vi "CFTS-Init State.vi"(9 "Root folder":path, 10 "CFTS Version":string, 11 "Experiment State (in)":T1) -> (0 "error out":errorcluster, 3 "Experiment State (out)":T1)   [LabVIEW 2020]
doc: "Initializes ABI experiment state based on the specified experiment ID."
uses:
  CFTS-Experiment State.ctl
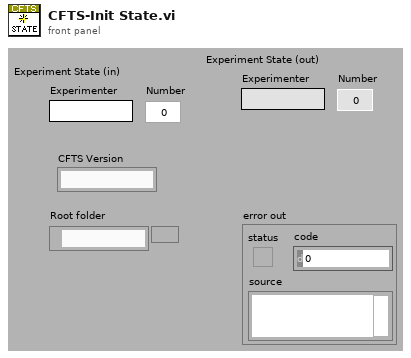
[diagram p1: front panel]
types:
  T1 = typedef "CFTS-Experiment State.ctl" = cluster{"Experimenter":string, "Number":u32, "Right":string, "Left":string, "Data Folder":path, "State File":path, "Version Info":string, "End Exposure Time":dbl, "Exposure Duration":string, "Run #":cluster{"CAP":i16, "ABR":i16, "DP":i16, "VsEP":i16, "MeasSeq":i16, "SubSeq":i16, "SFOAE":i16}}
  T2 = cluster{"CAP":i16, "ABR":i16, "DP":i16, "VsEP":i16, "MeasSeq":i16, "MeasSeq 2":i16, "MeasSeq 3":i16}
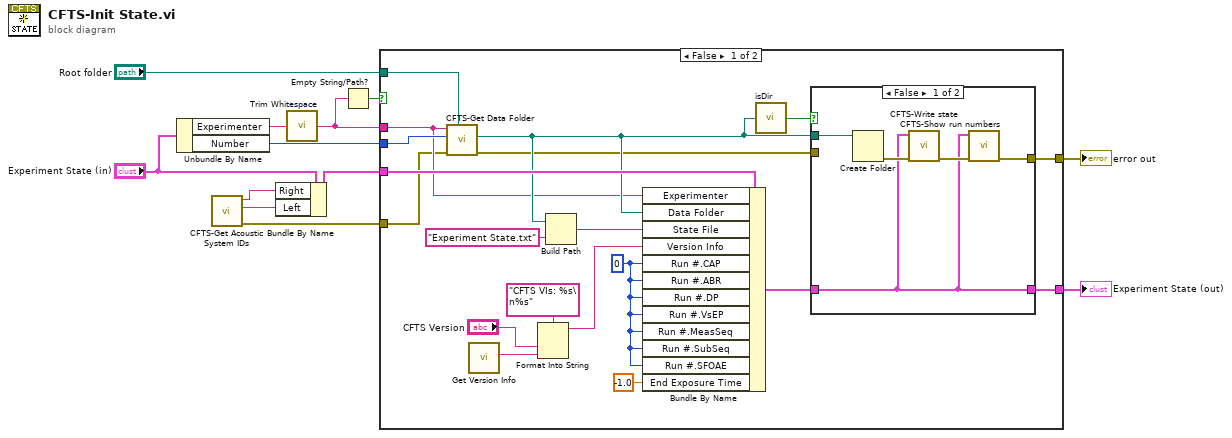
[diagram p0: block diagram]
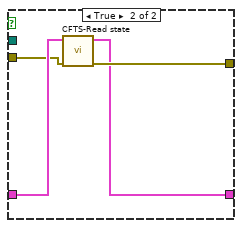
[diagram p2: hidden frame]
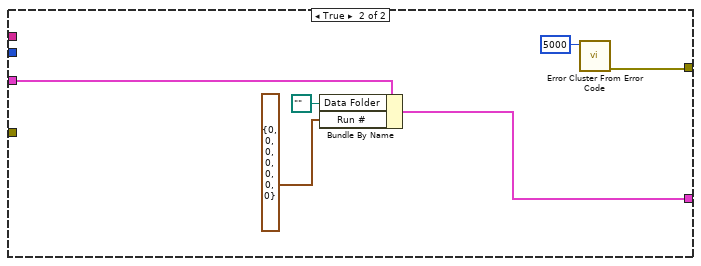
[diagram p3: hidden frame]
diagram:
  n1 = Unbundle By Name("Experiment State (in)") -> ("Experimenter"=w9:string, "Number"=w12:u32)
  n2 = call "CFTS-Get Acoustic System IDs.vi"() -> ("error out"=w2:errorcluster, "Left"=w6:string, "Right"=w5:string)  [unwired: 9 in]
  n3 = Bundle By Name(cluster="Experiment State (in)", "Right"=w5, "Left"=w6) -> (w3:T1)
  n4 = call <vilib>:"Trim Whitespace.vi"("string"=w9) -> ("trimmed string"=w8:string)  [unwired: 1 in]
  n5 = Empty String/Path?(string/path=w8) -> (empty?=w10:bool)
  n6 = case shown="False" w10 {
    tunnel: w3 -> [w31 w46]
    tunnel: [w18 w43] -> w7
    tunnel: w8 -> [w19 _]
    tunnel: w12 -> [w22 _]
    tunnel: [w17 w45] -> w11
    tunnel: w2 -> [w15 _]
    tunnel: "Root folder" -> [w13 _]
    frame False {
      w14 = u32 0 ("Next run #")
      n7 = call "CFTS-Get Data Folder.vi"("Root folder"=w13, "error in (no error)"=w15, "Number"=w22, "Experimenter"=w19) -> ("error out"=w16:errorcluster, "Data folder"=w24:path)  [unwired: 6 in]
      n8 = call "Get Version Info.vi"() -> ("Version Info"=w26:string)  [unwired: 10 in, 1 out]
      n9 = Format Into String(format string="CFTS VIs: %s\n%s", "CFTS Version", w26) -> (resulting string=w27:string)  [unwired: 2 in, 1 out]
      n10 = Build Path(base path=w24, name or relative path="Experiment State.txt") -> (appended path=w29:path)
      n11 = Bundle By Name(cluster=w31, "Experimenter"=w19, "Data Folder"=w24, "State File"=w29, "Version Info"=w27, "Run #.CAP"=w14, "Run #.ABR"=w14, "Run #.DP"=w14, "Run #.VsEP"=w14, "Run #.MeasSeq"=w14, "Run #.SubSeq"=w14, "Run #.SFOAE"=w14, "End Exposure Time"=-1.0) -> (w23:T1)
      n12 = call "isDir.vi"("path"=w24) -> ("is Dir?"=w25:bool)
      n13 = case shown="False" w25 {
        tunnel: w24 -> [w36 _]
        tunnel: [w33 w39] -> w18
        tunnel: w23 -> [w32 w40]
        tunnel: [w32 w38] -> w17
        tunnel: w16 -> [_ w37]
        frame False {
          n14 = Create Folder(path (use dialog)=w36) -> (error out=w35:errorcluster)  [unwired: 2 in, 2 out]
          n15 = call "CFTS-Write state.vi"("error in (no error)"=w35, "Experiment info"=w32) -> ("error out"=w34:errorcluster)  [unwired: 9 in]
          n16 = call "CFTS-Show run numbers.vi"("error in (no error)"=w34, "Expt State"=w32) -> ("error out"=w33:errorcluster)  [unwired: 9 in]
        }
        frame True {
          n17 = call "CFTS-Read state.vi"("error in (no error)"=w37, "Experiment info"=w40) -> ("error out"=w39:errorcluster, "Experiment info out"=w38:T1)  [unwired: 8 in]
        }
      }
    }
    frame True {
      n18 = Bundle By Name(cluster=w46, "Data Folder"=path "", "Run #"=T2 {"CAP"=0, "ABR"=0, "DP"=0, "VsEP"=0, "MeasSeq"=0, "MeasSeq 2"=0, "MeasSeq 3"=0}) -> (w45:T1)
      n19 = call <vilib>:"Error Cluster From Error Code.vi"("error code (0)"=5000) -> ("error out"=w43:errorcluster)  [unwired: 8 in]
    }
  }
  "Experiment State (out)" <- w11
  "error out" <- w7
